vi "Get Input.vi"() -> (3 "Input":string)   [LabVIEW 2021, in "AOC.lvlib"]
uses:
  AOC.lvlib
  <vilib>/Utility/error.llb/whitespace.ctl
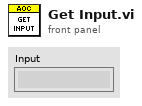
[diagram p1: front panel]
types:
  T1 = typedef "whitespace.ctl" = u16
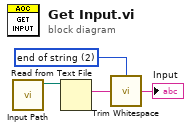
[diagram p0: block diagram]
diagram:
  w1 = T1 2 items=["both", "start of string", "end of string"] ("location (both)")
  n1 = call "Input Path.vi"() -> ("input path"=w4:path)  [unwired: 11 in]
  n2 = Read from Text File(file (use dialog)=w4) -> (text=w3:string)  [unwired: 3 in, 3 out]
  n3 = call <vilib>:"Trim Whitespace.vi"("string"=w3, "location (both)"=w1) -> ("trimmed string"=→"Input":string)
